vi "Open Index File.vi"(11 "file path (dialog if empty)":path) -> (3 "Array of points":string[][](array[string]))   [LabVIEW 2011]
uses:
  <vilib>/Utility/file.llb/Read From Spreadsheet File (string).vi
panel:
  out "all rows":string[][](array[string])
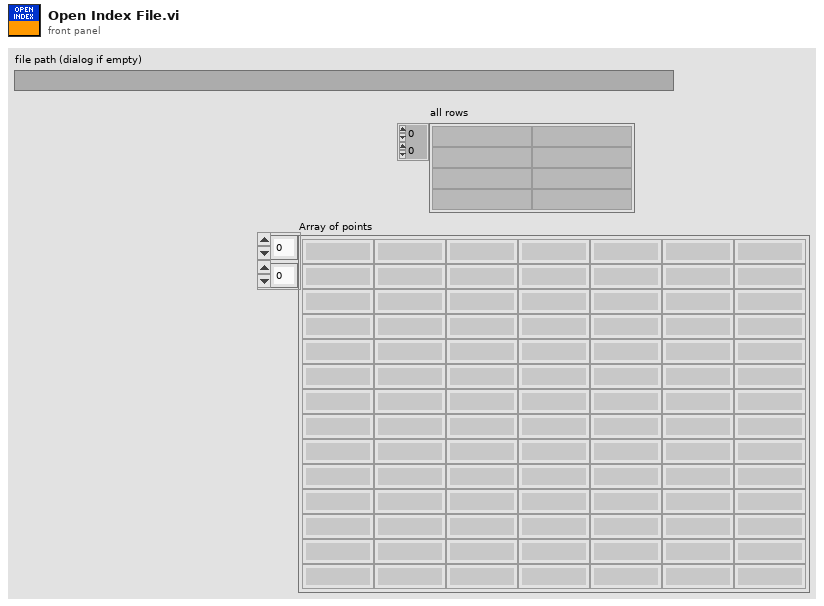
[diagram p1: front panel]
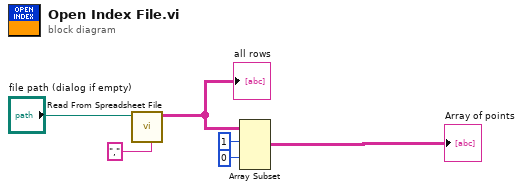
[diagram p0: block diagram]
diagram:
  n1 = call-poly <vilib>:"Read From Spreadsheet File.vi"("delimiter (\\t)"="," ("delimiter (\\t)"), "file path (dialog if empty)"="file path (dialog if empty)") -> ("all rows"=w5:string[][])  [unwired: 5 in, 4 out]
  "all rows" <- w5
  n2 = Array Subset(array=w5, index (row)=1 ("index"), index (col)=0 ("index")) -> (→"Array of points":string[][])  [unwired: 2 in]
